vi "Copy_Image_Greyscale_Mask_ARGB.vi"(8 "error in (no error)":errorcluster, 9 "Greyscale Image Mask":refnum<data-value>, 10 "ARGB Image Destination":refnum<data-value>, 11 "ARGB Image Source":refnum<data-value>) -> (0 "error out":errorcluster, 3 "ARGB Image Destination (duplicate)":refnum<data-value>)   [LabVIEW 2020, in "g_ar_toolkit.lvlib"]
uses:
  g_ar_toolkit.lvlib
  g_ar_toolkit.32.dll
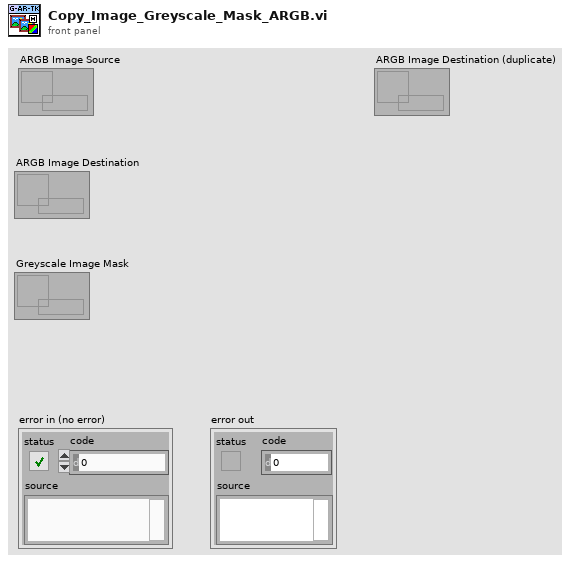
[diagram p1: front panel]
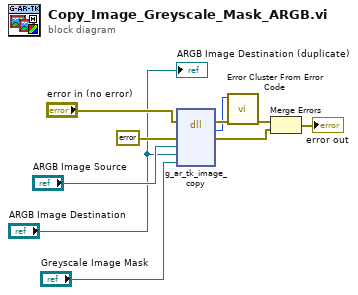
[diagram p0: block diagram]
diagram:
  n1 = dll-call lib="C:/serenial/libraries/g-augmented-reality-toolkit/LabVIEW/g_ar_toolkit/g_ar_toolkit.*.*" fn="g_ar_tk_image_copy"(error in="error in (no error)", "error_cluster"=errorcluster {"status"=FALSE, "code"=0, "source"=""} ("error constant"), "EDVR src"="ARGB Image Source", "EDVR dst"="ARGB Image Destination", "EDVR mask"="Greyscale Image Mask") -> (error out=w10:errorcluster, "MgErr"=w9:i32, "error_cluster"=w6:errorcluster)  [unwired: 5 in, 1 out]
  n2 = call <vilib>:"Error Cluster From Error Code.vi"("error in (no error)"=w10, "error code (0)"=w9) -> ("error out"=w8:errorcluster)  [unwired: 7 in]
  n3 = Merge Errors(w8, w6) -> (→"error out":errorcluster)
  "ARGB Image Destination (duplicate)" <- "ARGB Image Destination"
